vi "Init.vi"(8 "error in (no error)":errorcluster, 11 "BK-PSU in":refnum<class "BK-PSU.lvclass">) -> (0 "error out":errorcluster, 3 "BK-PSU out":refnum<class "BK-PSU.lvclass">)   [LabVIEW 2020, in "LAF2024Q2.lvlib" / "BK-PSU.lvclass"]
uses:
  BK-PSU.lvclass
  PowerSupplyVisa/PowerSupplyVisa.lvclass
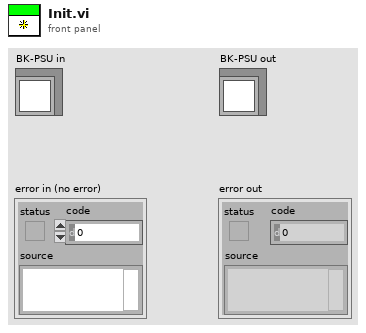
[diagram p1: front panel]
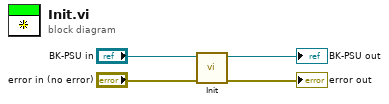
[diagram p0: block diagram]
diagram:
  n1 = call-parent "Init.vi"("error in (no error)"="error in (no error)", "PowerSupply in"="BK-PSU in") -> ("error out"=→"error out":errorcluster, "PowerSupply out"=→"BK-PSU out":refnum<class "BK-PSU.lvclass">)  [unwired: 8 in]
